vi "SubPanel_Oscilloscope_Block_Rev11_v2.vi"(2 "error input":errorcluster, 3 "Oscilloscope Configuration Input Array":T2(array[cluster]) {"vertical coupling" items=["AC", "DC", "Ground"]}) -> (0 "error out":errorcluster, 1 "Oscilloscope Configuration Output Array":T2(array[cluster]) {"vertical coupling" items=["AC", "DC", "Ground"]})   [LabVIEW 2019]
uses:
  Controls/OscilloscopeBlockControl.ctl
  <instrlib>/niScope/Controls/niScope vertical coupling.ctl
  <instrlib>/niScope/Configure/Trigger/niScope Configure Trigger Software.vi
panel:
  out "Oscilloscope Configuration Array Indicator":T2(array[cluster]) {"vertical coupling" items=["AC", "DC", "Ground"]}
  in  "Remove An Oscilloscope":bool
  in  "Oscilloscope Configuration Input Array":T3(array[cluster]) {"vertical coupling" items=["AC", "DC", "Ground"]}
  out "Horizontal:Actual Record Length":i32
  out "Configuration Errors":errorcluster
  in  "Oscilloscope Block Parameters":T4={"Oscilloscope"="", "channel names list"="", "vertical range"=10.0, "vertical coupling"=1, "Channel 0 50 ohms?"=FALSE, "50 ohm vertical range (V)"=10.0, "min record length"=1000, "min sample rate"=20000000.0} {"min sample rate" format="%^.2e"; "vertical coupling" items=["AC", "DC", "Ground"]}
  in  "EXIT SubVI":bool
  in  "Apply Configuration":bool
  # "Instructions\n\nSelect Oscilloscope Resource under \"Oscilloscope\"\n\nin a comma separate form (line 1, line 2, ...) type in the channel names of the device. \nIMPORTANT NOTE: \"line 1, line 2, ...\" will correspond to \"channel 0, channel 1, ...\" for each oscilloscope resource\n\nset the vertical range (no greater than 30)\n\nset the vertical coupling (dc) \n\nSet the channel 0 to 50 ohm impedance if you have something that requires 50 ohms to measure\n\nset 50 ohm vertical range if you have selected channel 0 50 ohms as true (ensure that it is no greater than 10\n\nmin record length (1000)\n\nmin sample rate (20e6) if you want a higher resolution, you increase the sample rate\n\npress apply configuration \n\nreview the instrument array above echoing your parameters created\n\nif you wish to remove a resource, select the oscilloscope resource in the \"oscillscope\" drop down\n\npress \"remove an oscilloscope\"\n\nonce fully configured, press \"EXIT\""
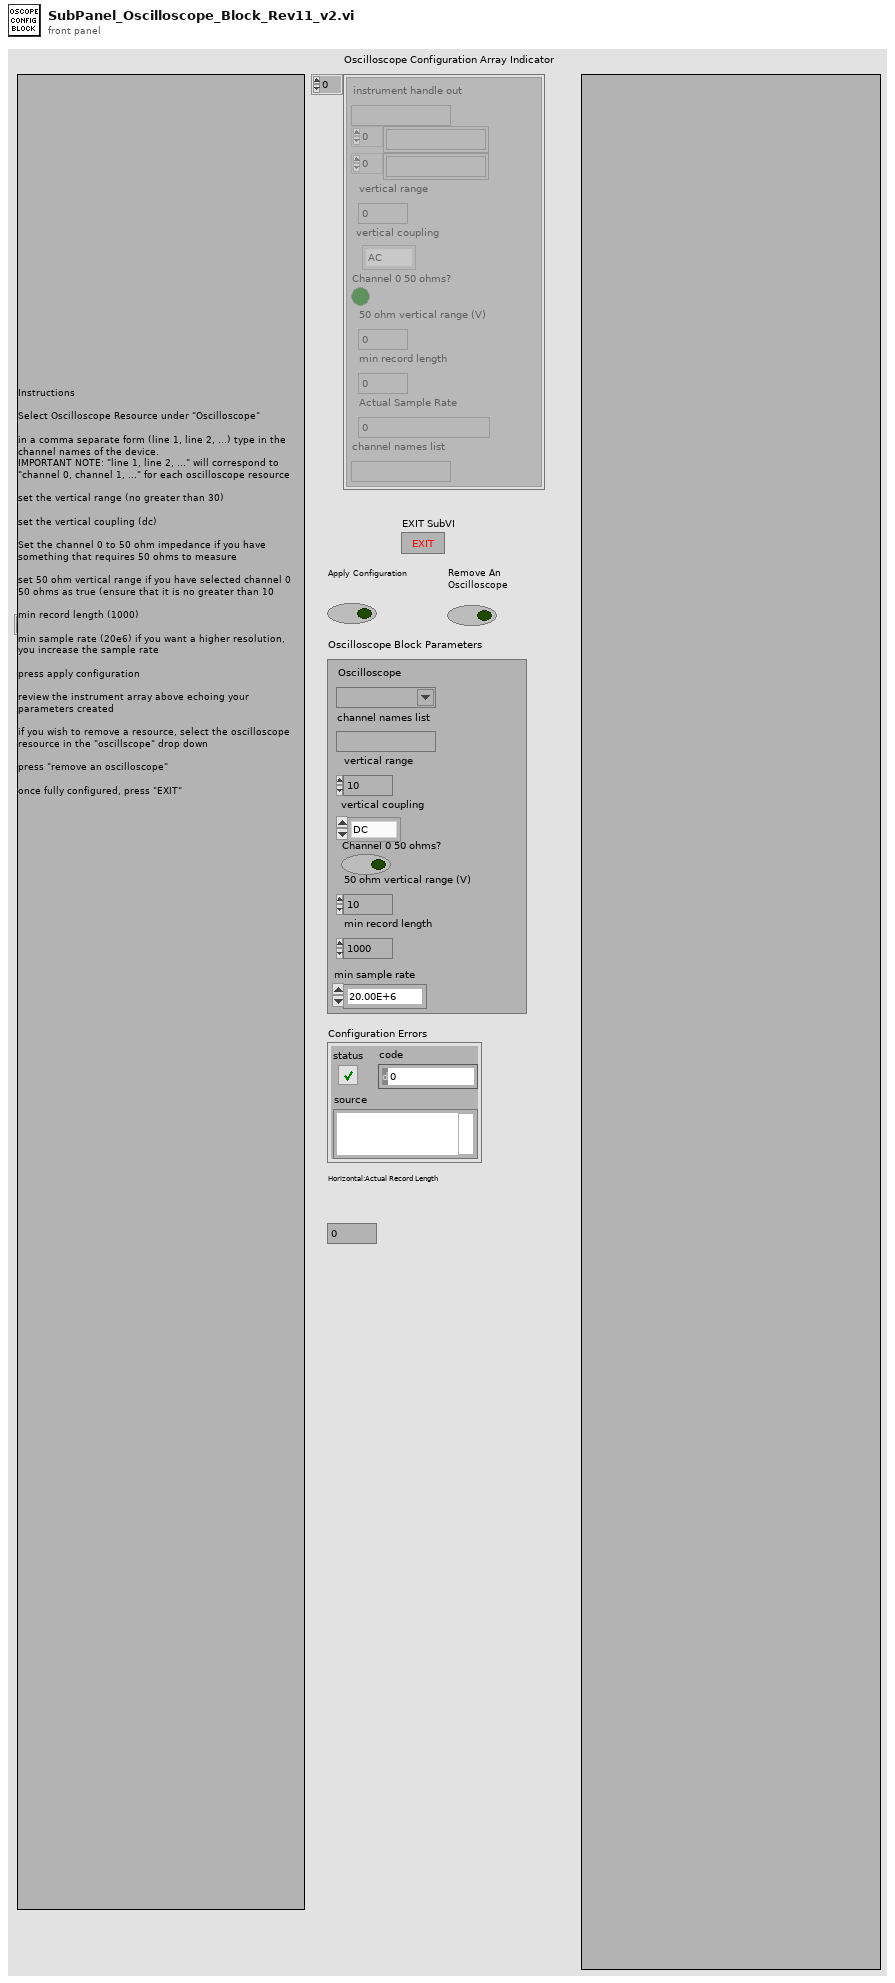
[diagram p1: front panel]
types:
  T1 = typedef "niScope vertical coupling.ctl" = i32
  T2 = cluster{"instrument handle out":refnum<k15>, string[], string[], "vertical range":dbl, "vertical coupling":T1, "Channel 0 50 ohms?":bool, "50 ohm vertical range (V)":dbl, "min record length":i32, "Actual Sample Rate":dbl, "channel names list":string}[]
  T3 = cluster{"instrument handle out":refnum<k15>, "channel numbers array":string[], "channel names array":string[], "vertical range":dbl, "vertical coupling":T1, "Channel 0 50 ohms?":bool, "50 ohm vertical range (V)":dbl, "min record length":i32, "Actual Sample Rate":dbl}[]
  T4 = typedef "OscilloscopeBlockControl.ctl" = cluster{"Oscilloscope":refnum<k15>, "channel names list":string, "vertical range":dbl, "vertical coupling":T1, "Channel 0 50 ohms?":bool, "50 ohm vertical range (V)":dbl, "min record length":i32, "min sample rate":dbl}
  T5 = cluster{"instrument handle out":refnum<k15>, string[], string[], "vertical range":dbl, "vertical coupling":T1, "Channel 0 50 ohms?":bool, "50 ohm vertical range (V)":dbl, "min record length":i32, "Actual Sample Rate":dbl, string}
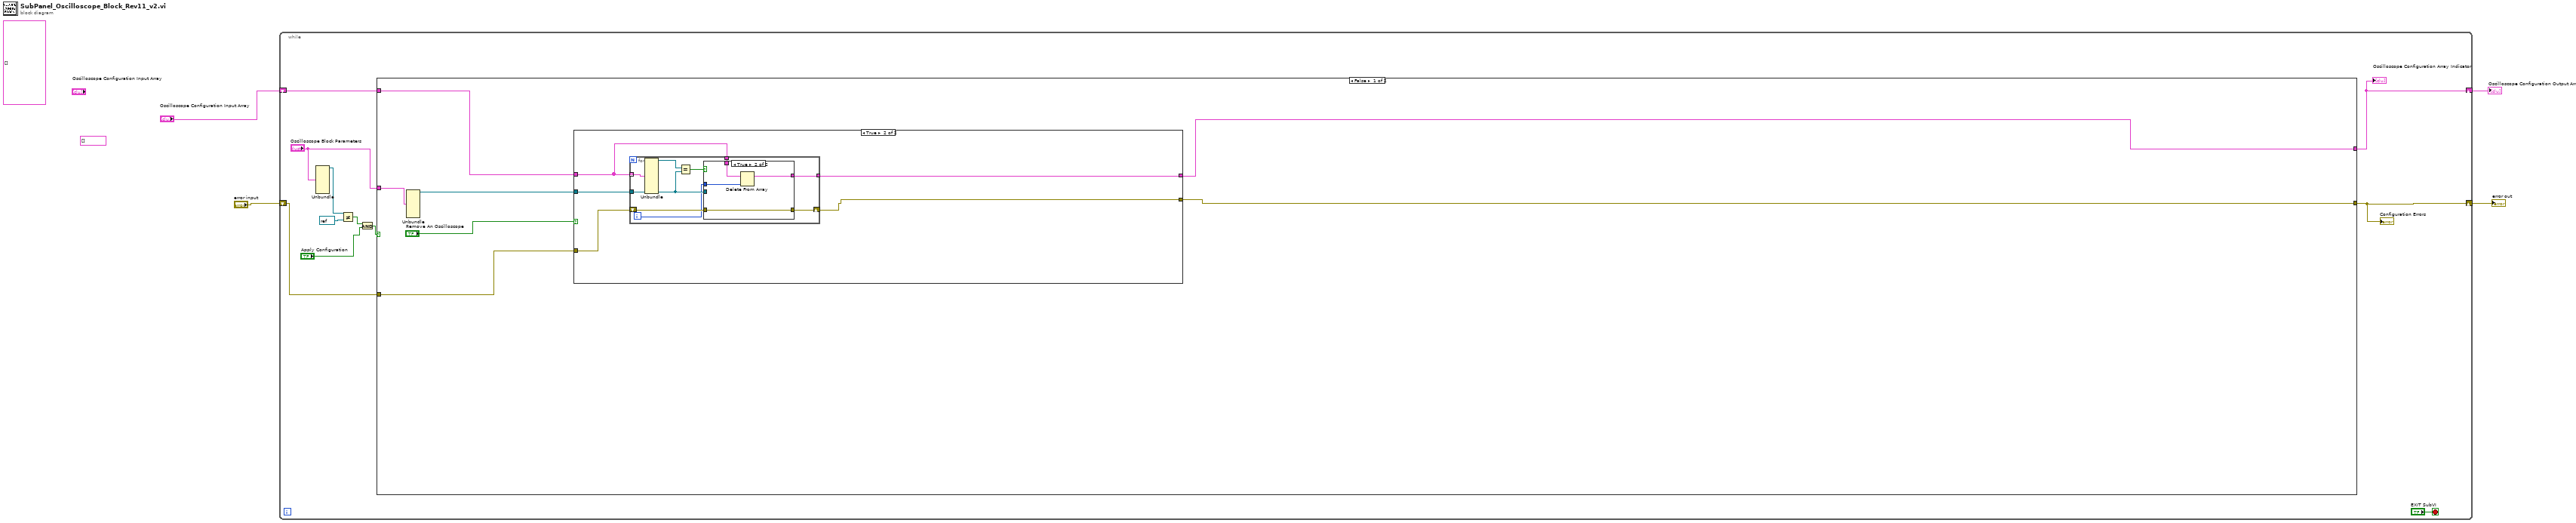
[diagram p0: block diagram]
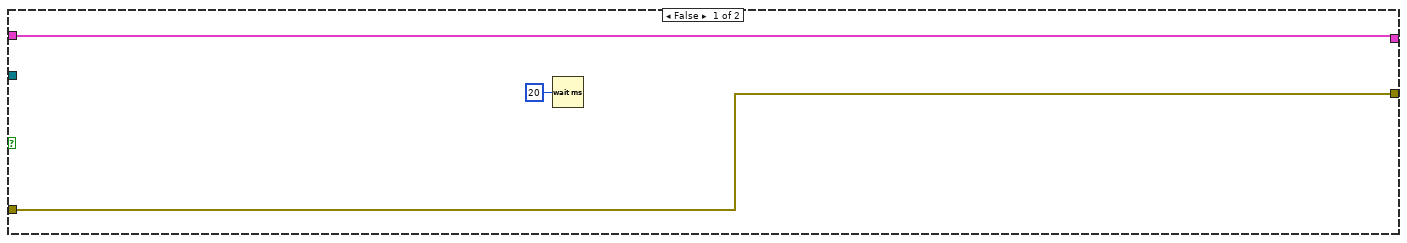
[diagram p2: hidden frame]
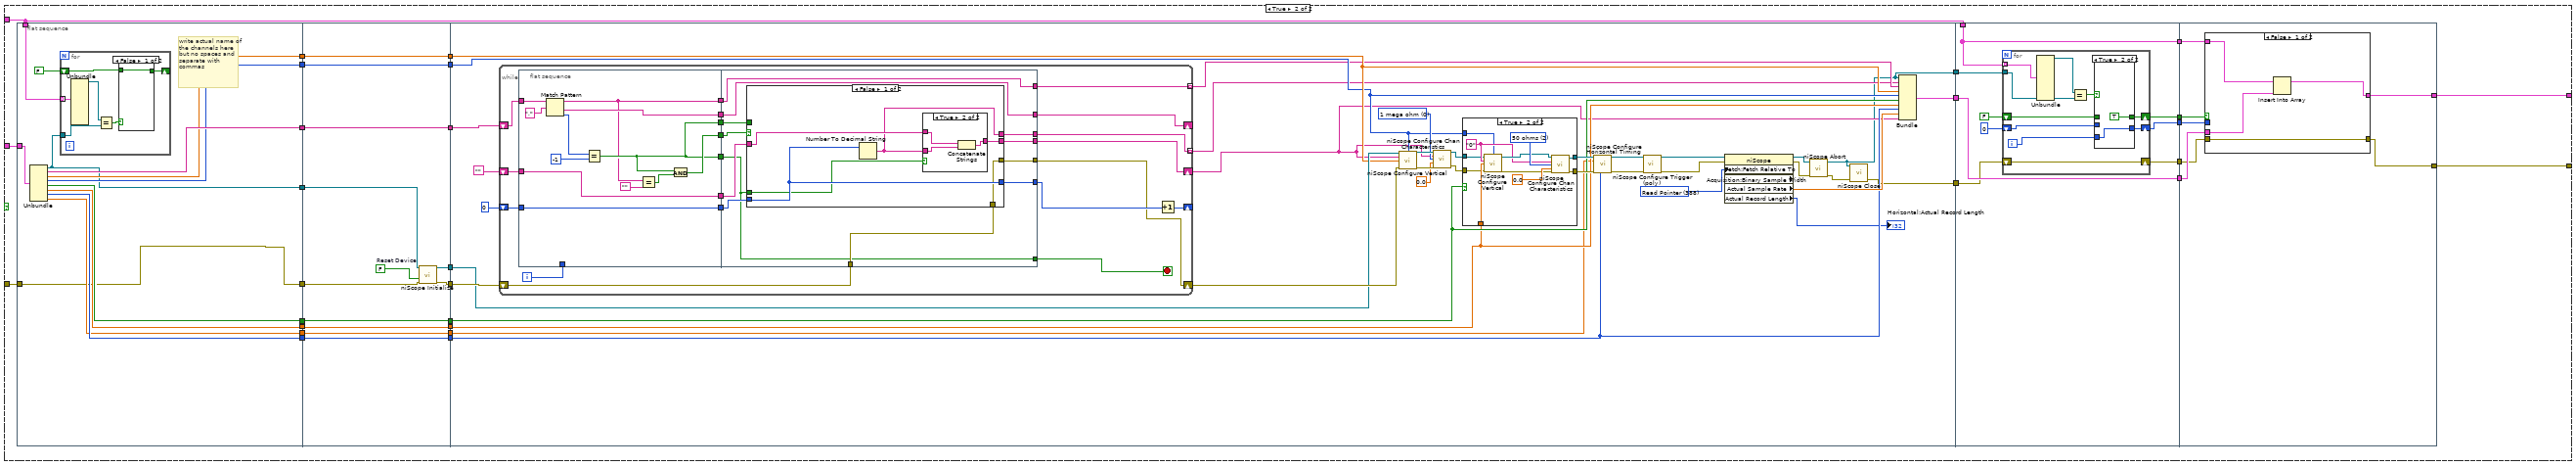
[diagram p4: hidden frame]
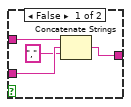
[diagram p6: hidden frame]
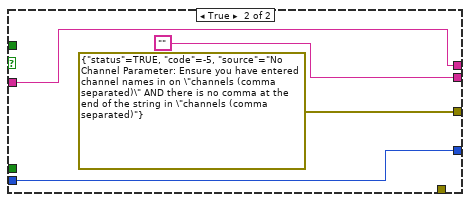
[diagram p7: hidden frame]
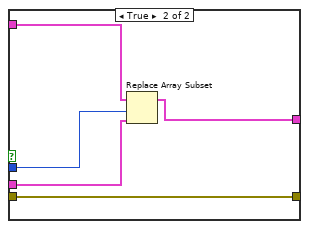
[diagram p10: hidden frame]
diagram:
  (unwired) T2 []
  (unwired) T3 [] ("Oscilloscope Configuration Input Array")
  n1 = while {
    shift-right: [w15] -> w4
    shift-left: "error input" -> [w13]
    shift-right: [w5] -> w1
    shift-left: "Oscilloscope Configuration Input Array" -> [w12]
    stop <- "EXIT SubVI" stop-if-true
    n2 = Unbundle("Oscilloscope Block Parameters") -> ("Oscilloscope"=w9:refnum<k15>)  [unwired: 7 out]
    n3 = Not Equal?(x=w9, y=refnum<k15> refnum ("resource name")) -> (x != y?=w8:bool)
    n4 = And(x=w8, y="Apply Configuration") -> (x .and. y?=w6:bool)
    n5 = case shown="False" w6 {
      tunnel: w13 -> [w19 w76]
      tunnel: [w18 w71] -> w15
      tunnel: [w16 w70] -> w5
      tunnel: w12 -> [w17 w46]
      tunnel: "Oscilloscope Block Parameters" -> [w22 w47]
      frame False {
        n6 = Unbundle(w22) -> ("Oscilloscope"=w20:refnum<k15>)  [unwired: 7 out]
        n7 = case shown="True" "Remove An Oscilloscope" {
          tunnel: w20 -> [_ w30]
          tunnel: w19 -> [w25 w29]
          tunnel: [w25 w26] -> w18
          tunnel: w17 -> [w23 w28]
          tunnel: [w23 w27] -> w16
          frame False {
            n8 = Wait (ms)(milliseconds to wait=u32 20) -> ()  [unwired: 1 out]
          }
          frame True {
            n9 = for {
              tunnel: w28 -> [w39] mode=indexing
              tunnel: w30 -> [w36]
              shift-right: [w34] -> w26
              shift-left: w29 -> [w35]
              tunnel: w28 -> [w33]
              tunnel: [w31] -> w27
              i -> [w32]
              n10 = Unbundle(w39) -> ("instrument handle out"=w38:refnum<k15>)  [unwired: 9 out]
              n11 = Equal?(x=w38, y=w36) -> (x = y?=w37:bool)
              n12 = case shown="True" w37 {
                tunnel: w36 -> [_ _]
                tunnel: w35 -> [w41 w42]
                tunnel: [w41 w42] -> w34
                tunnel: w33 -> [w40 w45]
                tunnel: w32 -> [_ w44]
                tunnel: [w40 w43] -> w31
                frame False {
                }
                frame True {
                  n13 = Delete From Array(array=w45, index=w44) -> (array with subset deleted=w43:T2)  [unwired: 1 in, 1 out]
                }
              }
            }
          }
        }
      }
      frame True {
        n14 = flat-sequence {
          tunnel: w76 -> [w77]
          tunnel: [w77] -> w72
          tunnel: [w79] -> w69
          tunnel: [w88] -> w68
          tunnel: [w87] -> w66
          tunnel: [w86] -> w64
          tunnel: [w85] -> w62
          tunnel: [w84] -> w60
          tunnel: [w83] -> w58
          tunnel: [w82] -> w56
          tunnel: w47 -> [w81]
          tunnel: w46 -> [w80]
          tunnel: [w104] -> w75
          tunnel: [w106] -> w74
          tunnel: [w105] -> w73
          tunnel: w72 -> [w107]
          tunnel: w69 -> [w103]
          tunnel: w68 -> [w104]
          tunnel: [w102] -> w67
          tunnel: w66 -> [w102]
          tunnel: [w101] -> w65
          tunnel: w64 -> [w101]
          tunnel: [w100] -> w63
          tunnel: w62 -> [w100]
          tunnel: [w99] -> w61
          tunnel: w60 -> [w99]
          tunnel: [w98] -> w59
          tunnel: w58 -> [w98]
          tunnel: [w97] -> w57
          tunnel: w56 -> [w97]
          tunnel: w73 -> [w127]
          tunnel: w74 -> [w130]
          tunnel: w75 -> [w117]
          tunnel: w67 -> [w126]
          tunnel: w65 -> [w125]
          tunnel: w63 -> [w124]
          tunnel: w61 -> [w123]
          tunnel: w59 -> [w122]
          tunnel: w57 -> [w121]
          tunnel: [w110] -> w55
          tunnel: [w128] -> w54
          tunnel: [w112] -> w53
          tunnel: w55 -> [w220]
          tunnel: w54 -> [w227]
          tunnel: w53 -> [w226]
          tunnel: w46 -> [w222]
          tunnel: [w219] -> w52
          tunnel: [w227] -> w51
          tunnel: [w223] -> w50
          tunnel: [w222] -> w49
          tunnel: [w221] -> w48
          tunnel: [w245] -> w70
          tunnel: [w242] -> w71
          tunnel: w52 -> [w243]
          tunnel: w51 -> [w244]
          tunnel: w50 -> [w248]
          tunnel: w49 -> [w247]
          tunnel: w48 -> [w246]
          frame #0 {
            # "write actual name of the channels here but no spaces and separate with commas"
            n15 = Unbundle(w81) -> ("Oscilloscope"=w79:refnum<k15>, "channel names list"=w88:string, "vertical range"=w87:dbl, "vertical coupling"=w86:T1, "Channel 0 50 ohms?"=w85:bool, "50 ohm vertical range (V)"=w84:dbl, "min record length"=w83:i32, "min sample rate"=w82:dbl)
            n16 = for {
              tunnel: w80 -> [w94] mode=indexing
              tunnel: w79 -> [w93]
              shift-right: [w90] -> _
              shift-left: FALSE -> [w89]
              n17 = Unbundle(w94) -> ("instrument handle out"=w92:refnum<k15>)  [unwired: 9 out]
              n18 = Equal?(x=w92, y=w93) -> (x = y?=w91:bool)
              n19 = case shown="False" w91 {
                selector: w91 -> [_ w96]
                tunnel: [w95 w96] -> w90
                tunnel: w89 -> [w95 _]
                frame False {
                }
                frame True {
                }
              }
            }
          }
          frame #1 {
            w108 = FALSE  # Reset Device
            n20 = call <instrlib>:"niScope Initialize.vi"("resource name"=w103, "reset device"=w108, "error in"=w107) -> ("instrument handle"=w105:refnum<k15>, "error out"=w106:errorcluster)  [unwired: 11 in]
          }
          frame #2 {
            w135 = 388 items=["Start"=482, "Trigger"=483, "Pretrigger"=477, "Now"=481, "Read Pointer"=388] ("Fetch:Fetch Relative To")
            w141 = u32 0 items=["1 mega ohm"=0, "50 ohms"=2] ("input impedance")
            n21 = while {
              shift-right: [w163] -> _
              shift-left: w117 -> [w164]
              shift-right: [w151] -> _
              shift-left: 0 -> [w156]
              shift-right: [w148] -> w116
              shift-left: "" -> [w154]
              tunnel: [w147] -> w120 mode=indexing
              shift-right: [w149] -> w144
              shift-left: w130 -> [w153]
              tunnel: [w145] -> w119 mode=indexing
              i -> [w162]
              stop <- w161 stop-if-true
              n22 = flat-sequence {
                tunnel: w164 -> [w174]
                tunnel: w162 -> [_]
                tunnel: [w172] -> w160
                tunnel: [w166] -> w159
                tunnel: [w167] -> w158
                tunnel: [w171] -> w157
                tunnel: w156 -> [w171]
                tunnel: [w170] -> w155
                tunnel: w154 -> [w170]
                tunnel: [w166] -> w150
                tunnel: [w165] -> w146
                tunnel: w160 -> [w188]
                tunnel: w159 -> [w179]
                tunnel: w158 -> [w187]
                tunnel: w157 -> [w185]
                tunnel: w155 -> [w184]
                tunnel: w153 -> [w183]
                tunnel: [w188] -> w163
                tunnel: [w179] -> w161
                tunnel: [w186] -> w148
                tunnel: [w182] -> w149
                tunnel: [w181] -> w152
                tunnel: w150 -> [w180]
                tunnel: [w178] -> w147
                tunnel: w146 -> [w178]
                tunnel: [w177] -> w145
                frame #0 {
                  n23 = Match Pattern(string=w174, regular expression=",") -> (before substring=w165:string, after substring=w172:string, offset past match=w176:i32)  [unwired: 1 in, 1 out]
                  n24 = Equal?(x=w176, y=-1) -> (x = y?=w166:bool)
                  n25 = Equal?(x=w165, y="") -> (x = y?=w168:bool)
                  n26 = And(x=w166, y=w168) -> (x .and. y?=w167:bool)
                }
                frame #1 {
                  n27 = case shown="False" w187 {
                    tunnel: [w190 ""] -> w186
                    tunnel: w185 -> [w194 w204]
                    tunnel: w184 -> [w192 w202]
                    tunnel: [w194 w204] -> w181
                    tunnel: w183 -> [w193 _]
                    tunnel: [w193 errorcluster {"status"=TRUE, "code"=-5, "source"="No Channel Parameter: Ensure you have entered channel names in on \"channels (comma separated)\" AND there is no comma at the end of the string in \"channels (comma separated)"} ("error out")] -> w182
                    tunnel: w180 -> [_ _]
                    tunnel: w179 -> [w191 _]
                    tunnel: [w189 w202] -> w177
                    frame False {
                      n28 = Number To Decimal String(number=w194) -> (decimal integer string=w189:string)  [unwired: 1 in]
                      n29 = case shown="True" w191 {
                        tunnel: w192 -> [w198 w201]
                        tunnel: w189 -> [w197 w200]
                        tunnel: [w195 w199] -> w190
                        frame False {
                          n30 = Concatenate Strings(w198, w197, "," ("string")) -> (w195:string)
                        }
                        frame True {
                          n31 = Concatenate Strings(w201, w200) -> (w199:string)
                        }
                      }
                    }
                    frame True {
                    }
                  }
                }
              }
              n32 = Increment(x=w152) -> (x+1=w151:i32)
            }
            n33 = call <instrlib>:"niScope Configure Vertical.vi"("instrument handle"=w127, "vertical coupling"=w125, "channels"=w116, "vertical range"=w126, "error in"=w144) -> ("instrument handle out"=w143:refnum<k15>, "error out"=w142:errorcluster)  [unwired: 9 in]
            n34 = call <instrlib>:"niScope Configure Chan Characteristics.vi"("instrument handle"=w143, "channels"=w116, "input impedance"=w141, "maximum input frequency"=0.0, "error in"=w142) -> ("instrument handle out"=w139:refnum<k15>, "error out"=w138:errorcluster)  [unwired: 9 in]
            n35 = case shown="True" w124 {
              tunnel: [w207 w218] -> w134
              tunnel: [w206 w217] -> w133
              tunnel: w123 -> [_ w211]
              tunnel: w139 -> [w207 w210]
              tunnel: w138 -> [w206 w209]
              tunnel: w125 -> [_ w208]
              frame False {
              }
              frame True {
                w215 = u32 2 items=["1 mega ohm"=0, "50 ohms"=2] ("input impedance")
                w212 = "0" ("channels")
                n36 = call <instrlib>:"niScope Configure Vertical.vi"("instrument handle"=w210, "vertical coupling"=w208, "channels"=w212, "vertical range"=w211, "error in"=w209) -> ("instrument handle out"=w214:refnum<k15>, "error out"=w213:errorcluster)  [unwired: 9 in]
                n37 = call <instrlib>:"niScope Configure Chan Characteristics.vi"("instrument handle"=w214, "channels"=w212, "input impedance"=w215, "maximum input frequency"=0.0, "error in"=w213) -> ("instrument handle out"=w218:refnum<k15>, "error out"=w217:errorcluster)  [unwired: 9 in]
              }
            }
            n38 = call <instrlib>:"niScope Configure Horizontal Timing.vi"("instrument handle"=w134, "min sample rate"=w121, "error in"=w133, "min record length"=w122) -> ("instrument handle out"=w137:refnum<k15>, "error out"=w136:errorcluster)  [unwired: 10 in]
            n39 = call-poly <instrlib>:"niScope Configure Trigger (poly).vi"("instrument handle"=w137, "error in"=w136) -> ("instrument handle out"=w115:refnum<k15>, "error out"=w114:errorcluster)  [unwired: 12 in]
            n40 = property class="niScope" props=["Fetch:Fetch Relative To", "Acquisition:Binary Sample Width", "Actual Sample Rate", "Actual Record Length"](reference=w115, error in=w114, "Fetch:Fetch Relative To"=w135) -> (reference out=w113:refnum<k15>, error out=w111:errorcluster, "Actual Sample Rate"=w129:dbl, "Actual Record Length"=→"Horizontal:Actual Record Length":i32)  [unwired: 1 out]
            n41 = call <instrlib>:"niScope Abort.vi"("instrument handle"=w113, "error in"=w111) -> ("instrument handle out"=w112:refnum<k15>, "error out"=w109:errorcluster)  [unwired: 12 in]
            n42 = call <instrlib>:"niScope Close.vi"("instrument handle"=w112, "error in"=w109) -> ("error out"=w110:errorcluster)  [unwired: 13 in]
            n43 = Bundle("instrument handle out"=w112, w119, w120, "vertical range"=w126, "vertical coupling"=w125, "Channel 0 50 ohms?"=w124, "50 ohm vertical range (V)"=w123, "min record length"=w122, "Actual Sample Rate"=w129, w116) -> (w128:T5)  [unwired: 1 in]
          }
          frame #3 {
            n44 = for {
              tunnel: w222 -> [w237] mode=indexing
              tunnel: w226 -> [w235]
              shift-right: [w232] -> w223
              shift-left: FALSE -> [w233]
              shift-right: [w230] -> w221
              shift-left: 0 -> [w231]
              shift-right: [w228] -> w219
              shift-left: w220 -> [w228]
              i -> [w229]
              n45 = Unbundle(w237) -> ("instrument handle out"=w236:refnum<k15>)  [unwired: 9 out]
              n46 = Equal?(x=w236, y=w235) -> (x = y?=w234:bool)
              n47 = case shown="True" w234 {
                tunnel: w233 -> [w239 _]
                tunnel: [w239 TRUE] -> w232
                tunnel: w231 -> [w238 _]
                tunnel: [w238 w240] -> w230
                tunnel: w229 -> [_ w240]
                frame False {
                }
                frame True {
                }
              }
            }
          }
          frame #4 {
            n48 = case shown="False" w248 {
              tunnel: w247 -> [w252 w257]
              tunnel: w244 -> [w251 w256]
              tunnel: w246 -> [_ w255]
              tunnel: [w250 w254] -> w245
              tunnel: [w249 w253] -> w242
              tunnel: w243 -> [w249 w253]
              frame False {
                n49 = Insert Into Array(array=w252, new element=w251) -> (w250:T2)  [unwired: 1 in]
              }
              frame True {
                n50 = Replace Array Subset(array=w257, new element=w256, index=w255) -> (w254:T2)
              }
            }
          }
        }
      }
    }
    "Configuration Errors" <- w15
    "Oscilloscope Configuration Array Indicator" <- w5
  }
  "error out" <- w4
  "Oscilloscope Configuration Output Array" <- w1
